vi "PV_Dlg_model.vi"() -> ()   [LabVIEW 2020]
doc: "Fonction :\n\nCe modèle peut être intégré très facilement à un subpannel à l'aide des fonctions de la palette Code Template >> Dynamic VI and Subpanel de la VIBOX"
panel:
  out "Stop<user event>":refnum<user-event>
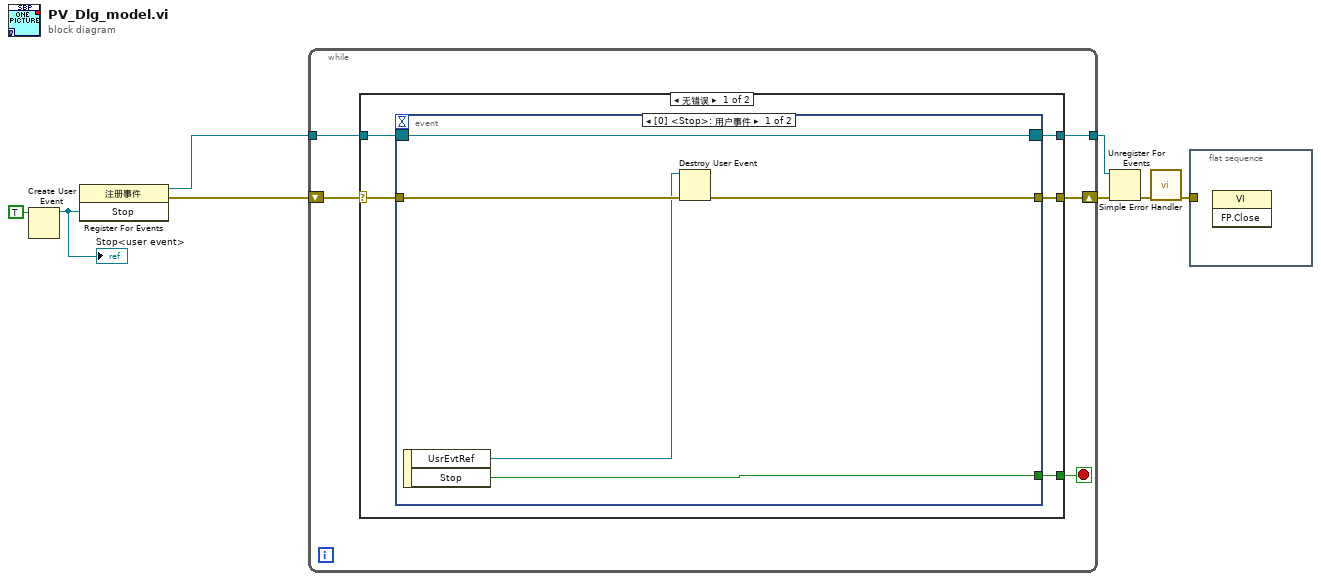
[diagram p0: block diagram]
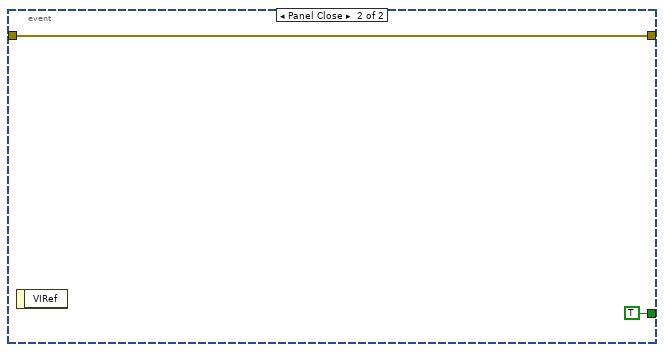
[diagram p2: hidden frame]
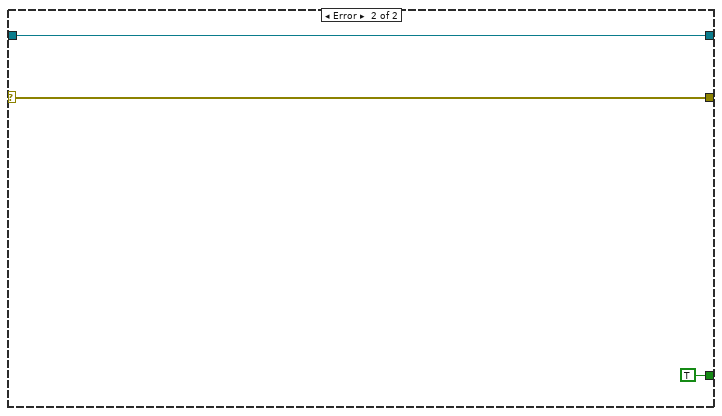
[diagram p3: hidden frame]
diagram:
  n1 = Create User Event(user event datatype=TRUE ("Stop")) -> (user event=w6:refnum<user-event>)  [unwired: 1 in, 1 out]
  "Stop<user event>" <- w6
  n2 = register-events(w6) -> (reference out=w5:refnum<event-registration>, error out=w1:errorcluster)  [unwired: 2 in]
  n3 = while {
    tunnel: w5 -> [w10]
    tunnel: [w9] -> w8
    shift-right: [w12] -> w4
    shift-left: w1 -> [w13]
    stop <- w11 stop-if-true
    n4 = case shown="无错误" w13 {
      selector: w13 -> [w15 w27]
      tunnel: [w14 w27] -> w12
      tunnel: [w16 TRUE] -> w11
      tunnel: w10 -> [w17 w26]
      tunnel: [w18 w26] -> w9
      frame No Error {
        n5 = event shown="[0] <Stop>: 用户事件" {
          selector: w17 -> [w23 _]
          dyn-events: [w23 _] -> w18
          timeout: _ -> [_ _]
          tunnel: [w20 TRUE ("Stop")] -> w16
          tunnel: w15 -> [w22 w24]
          tunnel: [w19 w24] -> w14
          event User Event {
            n6 = event-data() -> ("UsrEvtRef"=w21:refnum<user-event>, "Stop"=w20:bool)  [unwired: 1 out]
            n7 = Destroy User Event(user event=w21, error in=w22) -> (error out=w19:errorcluster)
          }
          event Panel Close {
            n8 = event-data() -> ()  [unwired: 2 out]
          }
        }
      }
      frame Error {
      }
    }
  }
  n9 = Unregister For Events(event registration refnum=w8, error in=w4) -> (error out=w7:errorcluster)
  n10 = call <vilib>:"Simple Error Handler.vi"("error in (no error)"=w7) -> ("error out"=w2:errorcluster)  [unwired: 1 in, 7 out]
  n11 = flat-sequence {
    tunnel: w2 -> [_]
    frame #0 {
      n12 = invoke class="VI" method="FP.Close"() -> ()  [unwired: 3 in, 3 out]
    }
  }
